vi "Query Inputs.vi"(8 "error in":errorcluster, 11 "PIOD in":refnum<class "PIOD.lvclass">) -> (0 "error out":errorcluster, 3 "PIOD out":refnum<class "PIOD.lvclass">)   [LabVIEW 2018, in "PIOD.lvlib" / "PIOD.lvclass"]
uses:
  PIOD.lvclass
  <vilib>/ethernetip/ethernetip.llb/EthernetIPSLC500FileType.ctl
  Custom Controls/File Number.ctl
  PIOD.lvclass/PIOD.ctl
  Accessors/Read/Read Timeout (ms).vi
  <vilib>/ethernetip/ethernetip.llb/EthernetIP SLC500 Read Raw.vi
  <vilib>/ethernetip/ethernetip.lvlib
  PPLs/PLC/Parent/PLC.lvlibp/PLC.lvclass
  C:/AME Test Engineering/LabVIEW/PPLs/PLC/Parent/PLC.lvlibp/PLC.lvclass
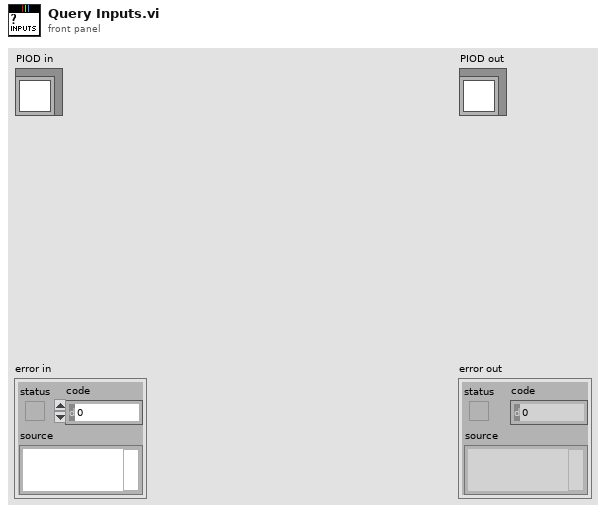
[diagram p1: front panel]
types:
  T1 = typedef "PIOD.lvlib/PIOD.lvclass/File Number.ctl" = enum16{"Output", "Input", "Status", "Output2"}
  T2 = typedef "ethernetip.lvlib/EthernetIPSLC500FileType.ctl" = u8
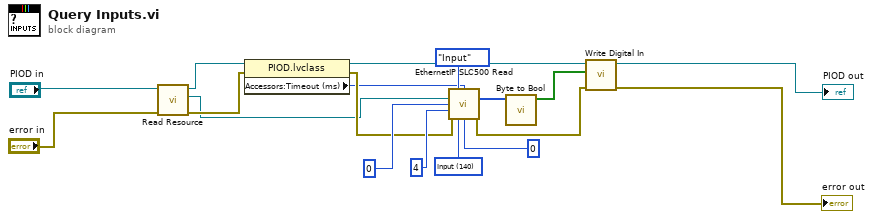
[diagram p0: block diagram]
diagram:
  w18 = T2 140 items=["Status"=132, "Bit"=133, "Timer"=134, "Counter"=135, "Control"=136, "Integer"=137, "Float"=138, "Output"=139, "Input"=140, "String"=141, "ASCII"=142] ("File Type")
  n1 = call "Read Resource.vi"("error in (no error)"="error in", "PLC in"="PIOD in") -> ("error out"=w9:errorcluster, "Resource"=w6:refnum<visa-resource-name>, "PLC out"=w7:refnum<class "PIOD.lvclass">)  [unwired: 7 in]
  n2 = property class="PIOD.lvclass"(reference=w7, error in=w9) -> (reference out=w5:refnum<class "PIOD.lvclass">, error out=w12:errorcluster, "Accessors:Timeout (ms)"=w11:i32)
  n3 = call-poly <vilib>:"EthernetIP SLC500 Read.vi"("File Number"=File_Number."Input", "Timeout (ms)"=w11, "Network Path"=w6, "Element Number"=u16 0, "Number of Bytes"=u32 4, "error in"=w12, "File Type"=w18, "Subelement Number"=u16 0) -> ("Data"=w13:u8[], "error out"=w2:errorcluster)  [unwired: 5 in, 1 out]
  n4 = call "Byte to Bool.vi"("Data In"=w13) -> ("Data out"=w4:bool[])  [unwired: 10 in]
  n5 = call "Write Digital In.vi"("error in (no error)"=w2, "Digital In"=w4, "PLC in"=w5) -> ("error out"=→"error out":errorcluster, "PLC out"=→"PIOD out":refnum<class "PIOD.lvclass">)  [unwired: 7 in]
